vi "Publish UI VI Ref.vi"(8 "error in (no error)":errorcluster, 10 "VI Ref":refnum<vi>, 11 "Flex UI (Actor) in":refnum<class "Flex UI (Actor).lvclass">) -> (0 "error out":errorcluster, 3 "Flex UI (Actor) out":refnum<class "Flex UI (Actor).lvclass">)   [LabVIEW 2016, in "Flex UI (Parent Actor).lvlib" / "Flex UI (Actor).lvclass"]
uses:
  Flex UI (Actor).lvclass
  <vilib>/East West Architects/MVC Subscription/Subscription/MVC Subscription.lvclass
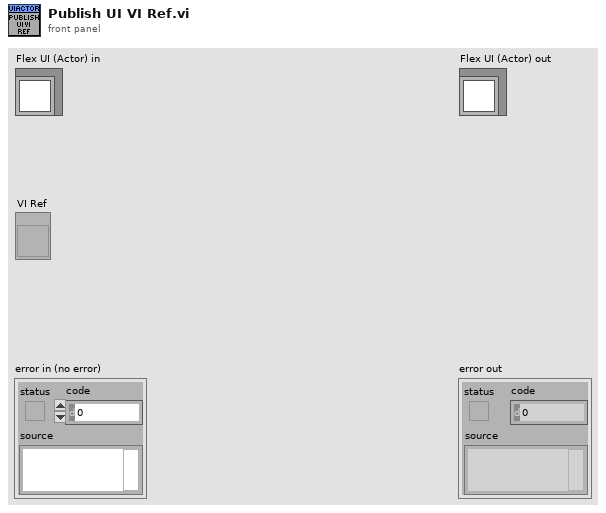
[diagram p1: front panel]
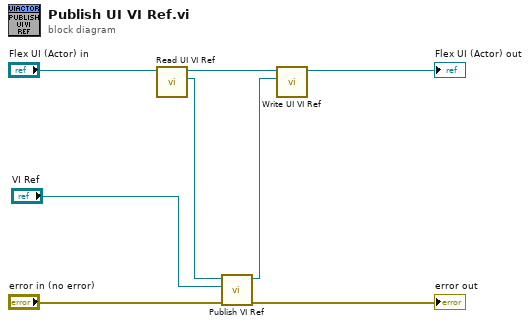
[diagram p0: block diagram]
diagram:
  n1 = call-dynamic "Read UI VI Ref.vi"("Flex UI (Actor) in"="Flex UI (Actor) in") -> ("UI VI Ref"=w2:refnum<class "MVC Subscription.lvclass">, "Flex UI (Actor) out"=w3:refnum<class "Flex UI (Actor).lvclass">)  [unwired: 9 in]
  n2 = call <vilib>:"Publish VI Ref.vi"("error in (no error)"="error in (no error)", "VI Ref"="VI Ref", "MVC Subscription in"=w2) -> ("error out"=→"error out":errorcluster, "MVC Subscription out"=w1:refnum<class "MVC Subscription.lvclass">)  [unwired: 7 in]
  n3 = call-dynamic "Write UI VI Ref.vi"("UI VI Ref"=w1, "Flex UI (Actor) in"=w3) -> ("Flex UI (Actor) out"=→"Flex UI (Actor) out":refnum<class "Flex UI (Actor).lvclass">)  [unwired: 9 in]
